vi "Dll_debug.vi"   [LabVIEW 2011]
uses:
  Certificate_01.vi
types:
  T1 = enum16{"Open", "Verify", "Password", "Log", "Close"}
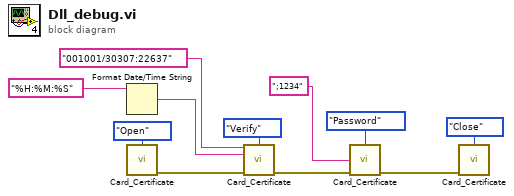
[diagram p0: block diagram]
diagram:
  n1 = Format Date/Time String(time format string (%c)="%H:%M:%S") -> (date/time string=w2:string)  [unwired: 2 in]
  n2 = call-poly "Card_Certificate.vi"("DB"=T1."Open") -> ("error out"=w7:errorcluster)  [unwired: 13 in, 1 out]
  n3 = call-poly "Card_Certificate.vi"("CardNumber"="001001/30307:22637", "DB"=T1."Verify", "Time"=w2, "error in"=w7) -> ("error out"=w6:errorcluster)  [unwired: 10 in, 1 out]
  n4 = call-poly "Card_Certificate.vi"("DB"=T1."Password", "Password"=";1234", "error in"=w6) -> ("error out"=w5:errorcluster)  [unwired: 11 in, 1 out]
  n5 = call-poly "Card_Certificate.vi"("DB"=T1."Close", "error in"=w5) -> ()  [unwired: 12 in, 2 out]
